vi "Main Core UI.vi"(8 "error in (no error)":errorcluster, 11 "Module_Refs":T5={"ModuleName"=enum."Controller", "Queue"=refnum, "user event"=refnum, "VI Refnum"=refnum, "ShowFP"=FALSE, "StatesTracking Enabled"=FALSE}) -> (0 "error out":errorcluster)   [LabVIEW 2021, in "Core UI.lvlib"]
doc: "Main Module Template of the architecture. Use this as a template to integrate new independent processes into your application."
uses:
  Core UI.lvlib
  Typedefs/Module References.ctl
  Typedefs/Enum_Module_Name.ctl
  Typedefs/Message.ctl
  GameEl_class/private/Enum Direction.ctl
  Application/Backgroud_v2.ctl
  Application/Shield.ctl
  Application/Grapes.ctl
  Typedefs/State Machine Data.ctl
  Typedefs/Config.ctl
  Configuration/Typedefs/App Cfg DVR.ctl
  Typedefs/Application Configuration.ctl
  Module Template/Typedefs/Config.ctl
  Modules/Sound Manager/Typedefs/Config.ctl
  Core UI Configuraton Extractor API.vi
  Configuration/Configuration.lvlib
  Architecture.lvlib
  Module Template/Module Template.lvlib
  Modules/Sound Manager/Sound Manager.lvlib
  GameEl_class/GameEl.lvclass
  Application/Application.lvclass
panel:
  out "Image Ring":u16(ring)
  out "Star":bool
  in  "Grapes":T1
  in  "Shield":T2
  in  "Studios":bool caption="Creator 2"
  in  "Creator":bool
  out "TIME":string
  out "SCORE":string
  out "Board Game":u32[][](array[colorbox])
  out "Background":T3=1
  in  "Usert Stop Game":bool
  in  "Pause/Resume":bool
  out "Direction":T4
  out "Current Score":u16
  in  "Stop App":bool
  out "Message":string
  in  "Stop Module":bool
  # "#Architecture\n\nPlace inside this box all visible data."
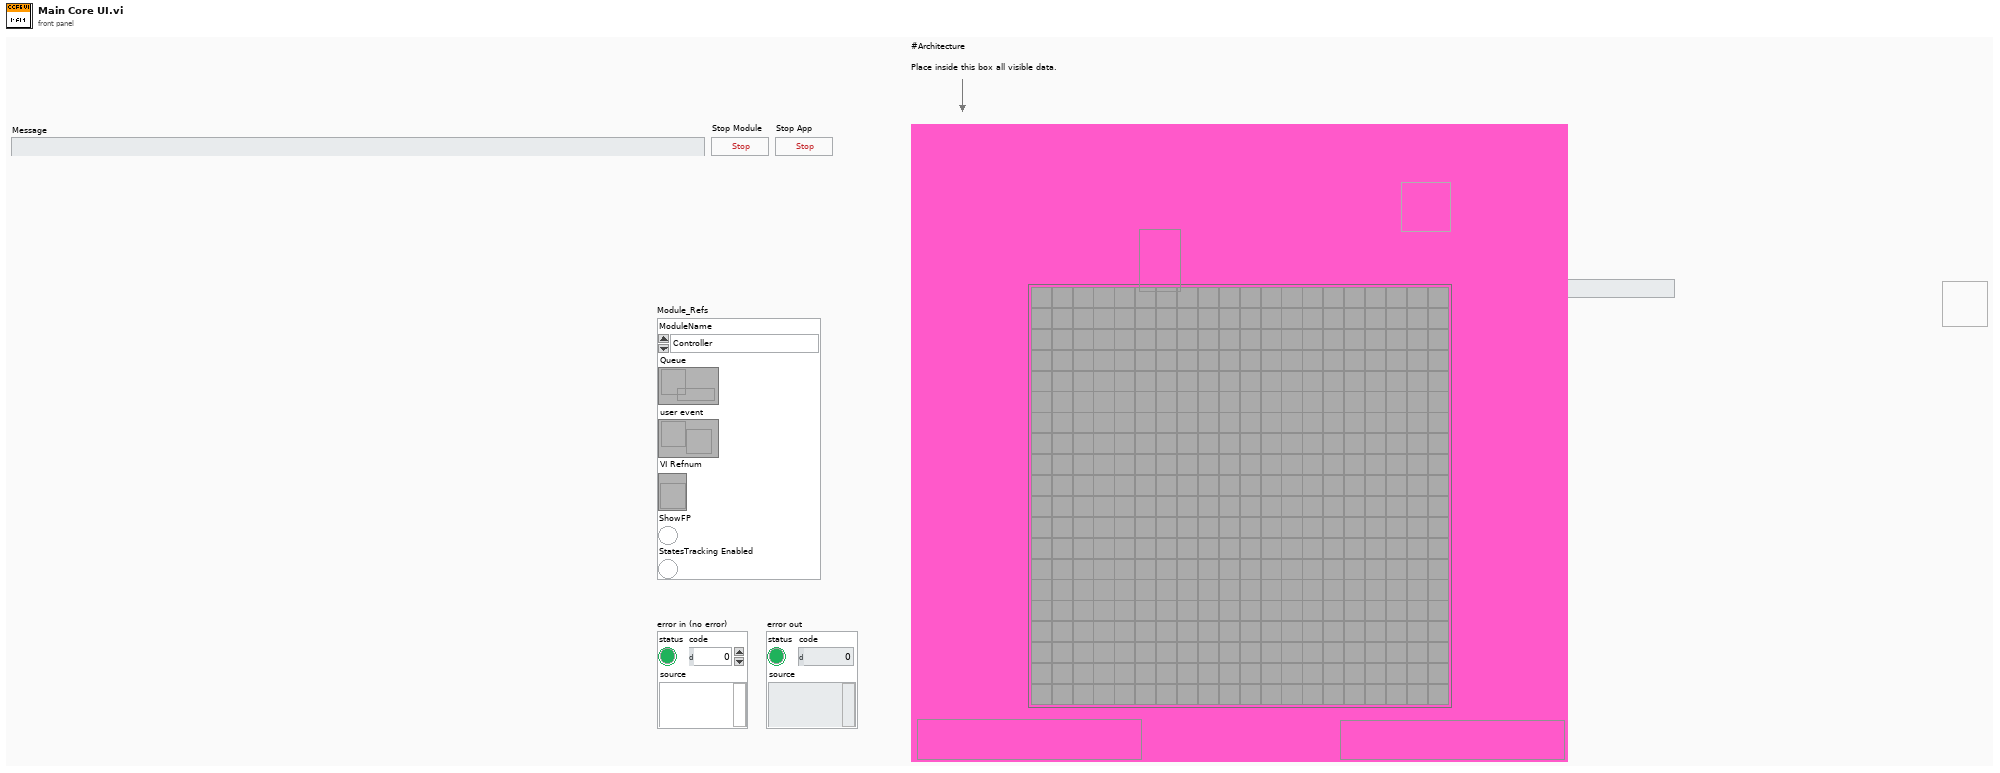
[diagram p1: front panel]
types:
  T1 = typedef "Application.lvclass/Grapes.ctl" = u16
  T2 = typedef "Application.lvclass/Shield.ctl" = u16
  T3 = typedef "Application.lvclass/Backgroud_v2.ctl" = u16
  T4 = typedef "GameEl.lvclass/Enum Direction.ctl" = enum16{"Up", "Down", "Forward", "Backward"}
  T5 = typedef "Architecture.lvlib/Module References.ctl" = cluster{"ModuleName":T6, "Queue":refnum<queue>, "user event":refnum<user-event>, "VI Refnum":refnum<vi>, "ShowFP":bool, "StatesTracking Enabled":bool}
  T6 = typedef "Configuration.lvlib/Enum_Module_Name.ctl" = enum16{"Configuration", "Error_Handler", "Log", "Database", "Controller", "UI Module", "Sound Manager"}
  T7 = typedef "Core UI.lvlib/State Machine Data.ctl" = cluster{"Module_Refs":T5, "Response Data":variant, "Core UI Config":T8}
  T8 = typedef "Core UI.lvlib/Config.ctl" = cluster{"Module Enabled":bool}
  T9 = enum32{"Invalid", "Standard", "Closed", "Hidden", "Minimized", "Maximized"}
  T10 = typedef "Error_Manager.lvlib/LogRotate.lvclass/LogData.ctl" = cluster{"error in":errorcluster, "replacements":string[], "Time Stamp":timestamp}
  T11 = typedef "Configuration.lvlib/App Cfg DVR.ctl" = refnum<data-value>
  T12 = typedef "Module Template.lvlib/Config.ctl" = cluster{"Module Enabled":bool}
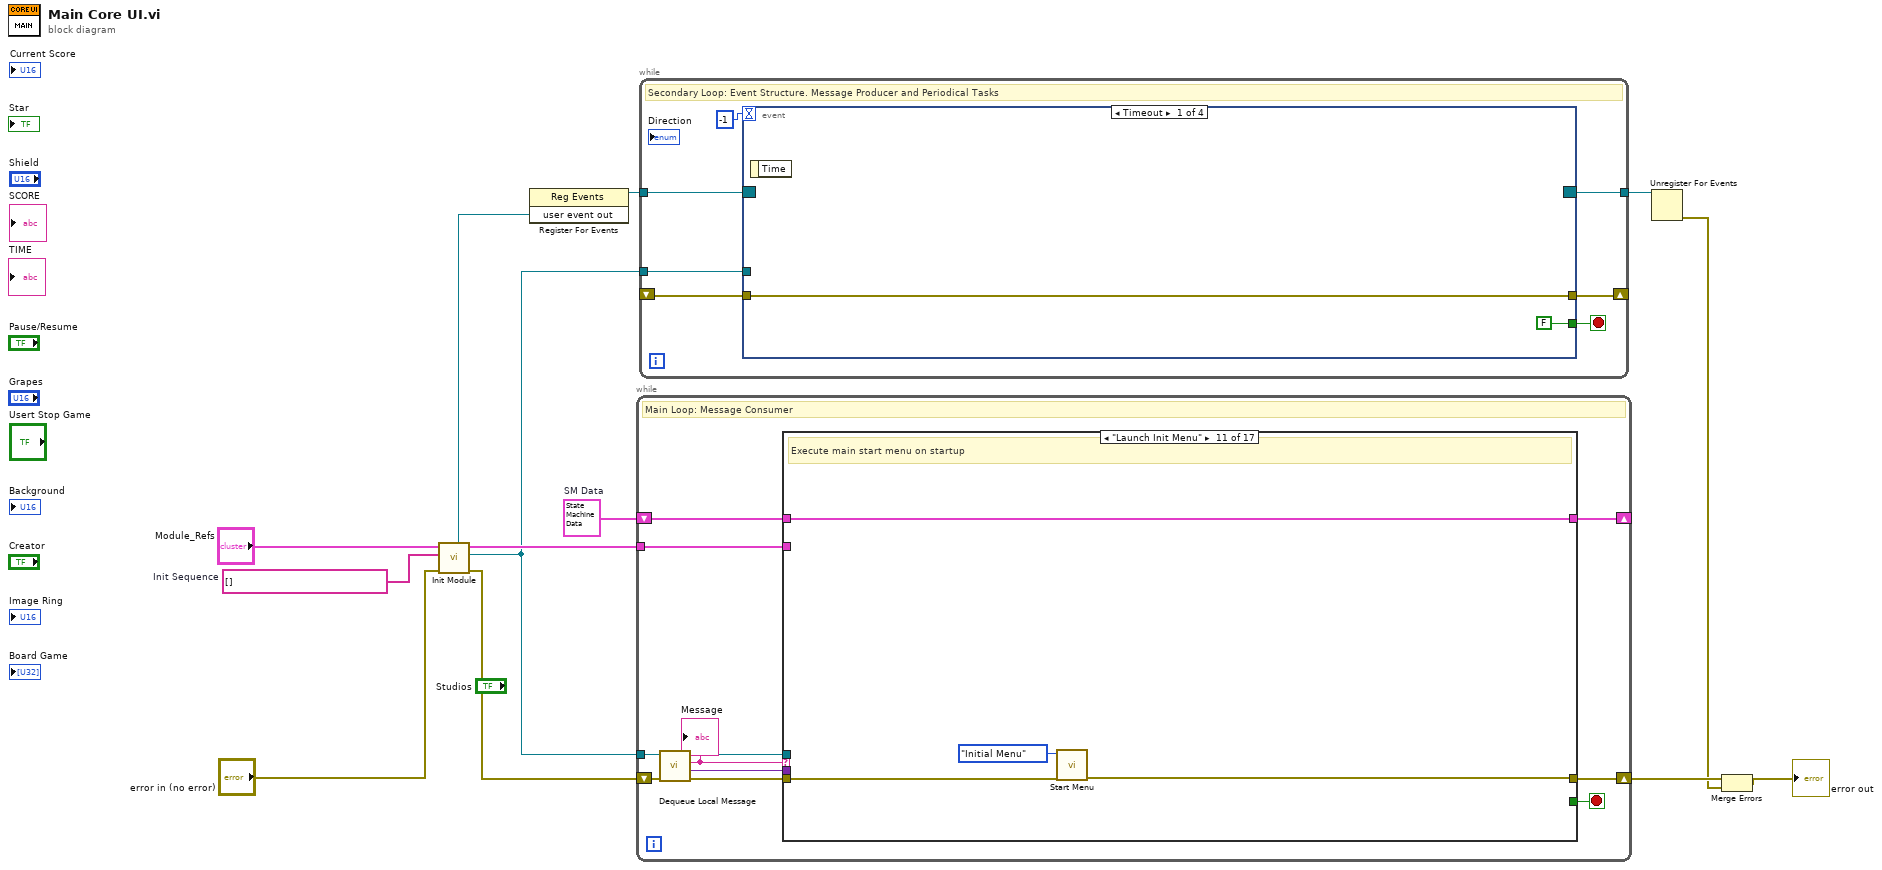
[diagram p0: block diagram]
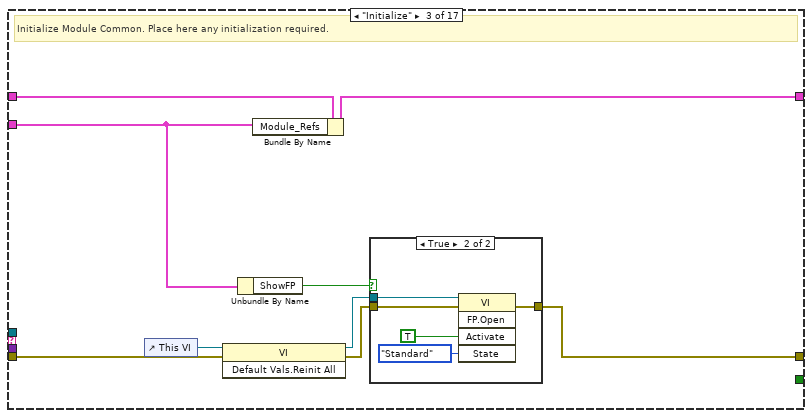
[diagram p4: hidden frame]
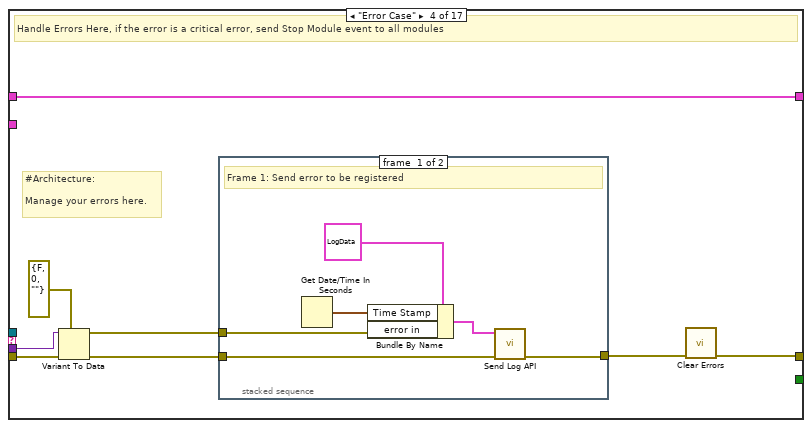
[diagram p6: hidden frame]
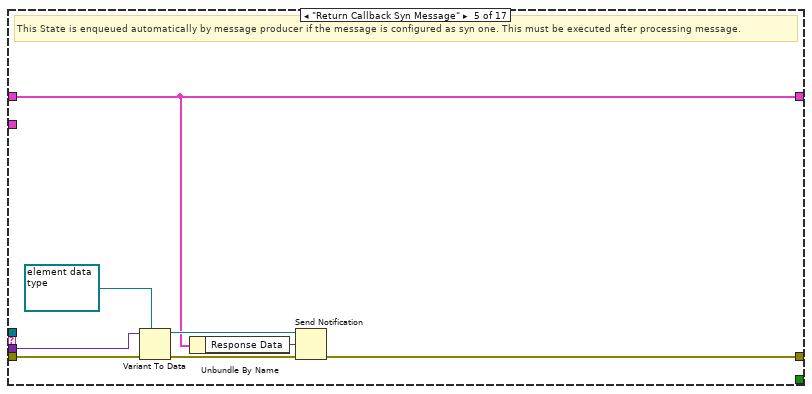
[diagram p9: hidden frame]
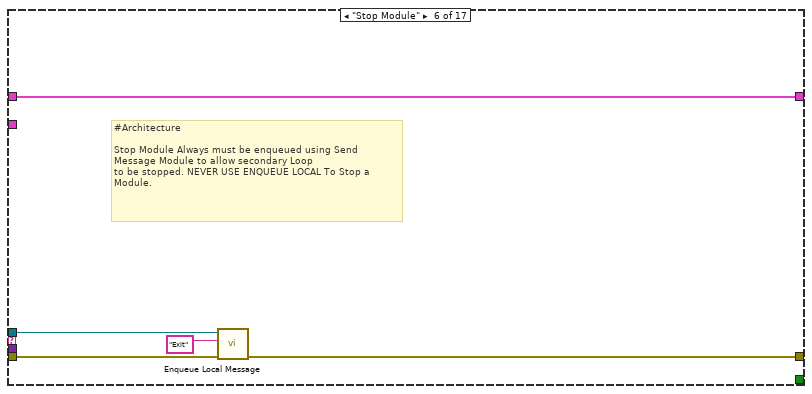
[diagram p10: hidden frame]
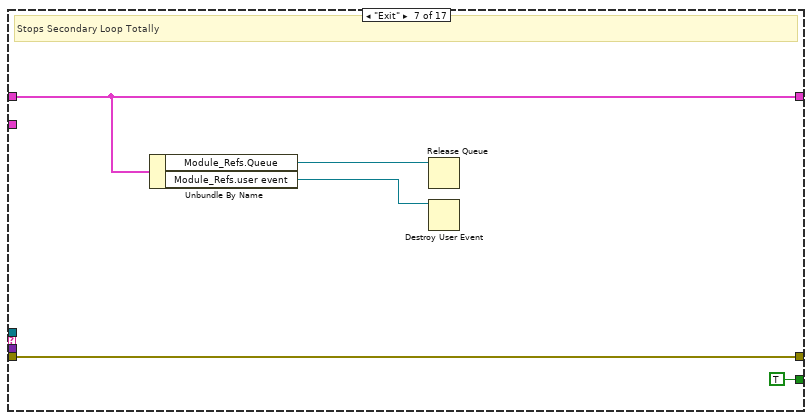
[diagram p11: hidden frame]
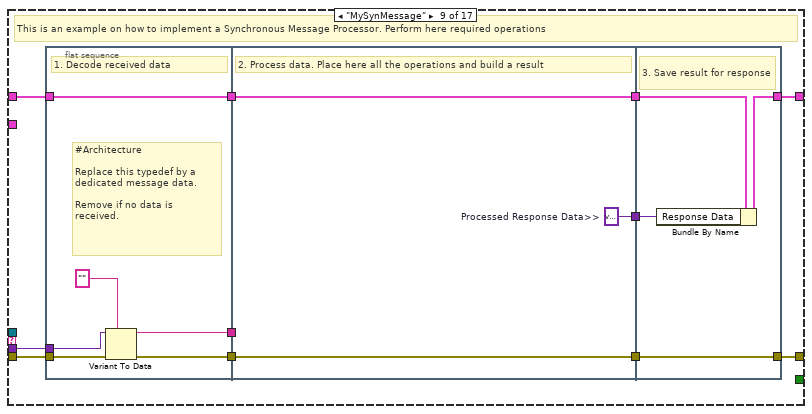
[diagram p13: hidden frame]
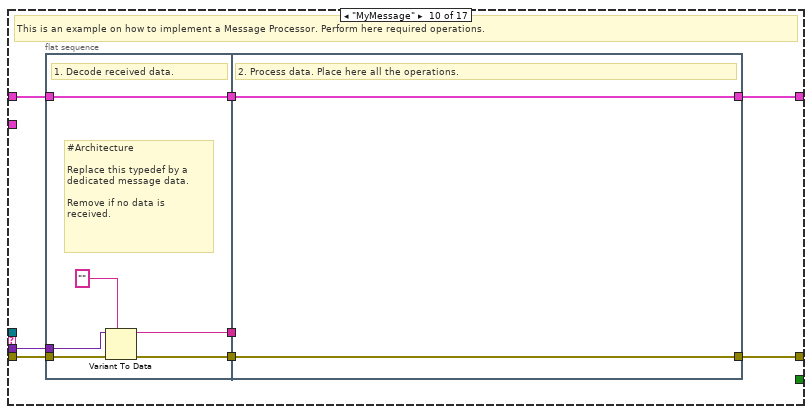
[diagram p14: hidden frame]
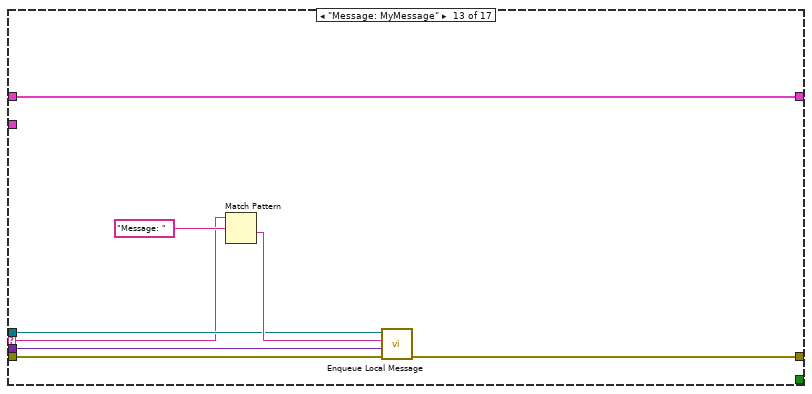
[diagram p16: hidden frame]
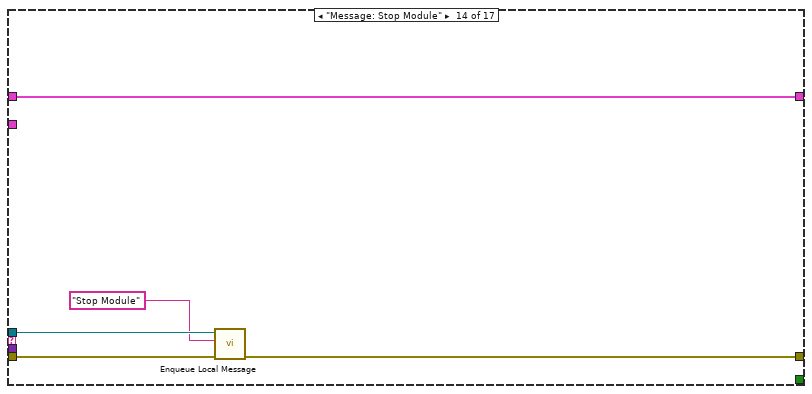
[diagram p17: hidden frame]
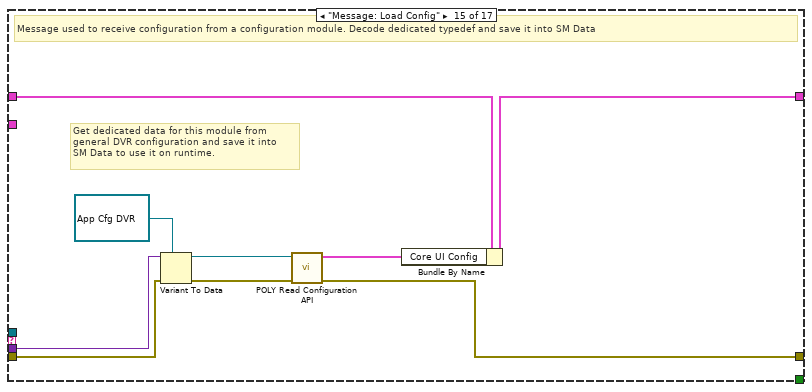
[diagram p18: hidden frame]
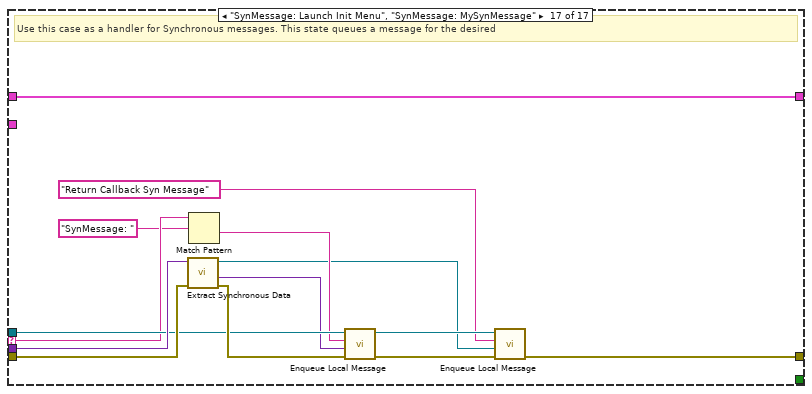
[diagram p20: hidden frame]
diagram:
  w10 = string[] []  # Init Sequence
  w13 = T7 {"Module_Refs"={"ModuleName"=enum."Controller", "Queue"=refnum, "user event"=refnum, "VI Refnum"=refnum, "ShowFP"=FALSE, "StatesTracking Enabled"=FALSE}, "Response Data"=variant, "Core UI Config"={"Module Enabled"=FALSE}}  # SM Data
  n1 = call "Init Module.vi"("error in (no error)"="error in (no error)", "Init Sequence"=w10, "Module Refs"="Module_Refs") -> ("error out"=w12:errorcluster, "queue out"=w1:refnum<queue>, "Module Refs Out"=w3:T5, "user event out"=w2:refnum<user-event>)  [unwired: 5 in]
  n2 = register-events(w2) -> (reference out=w9:refnum<event-registration>)  [unwired: 2 in, 1 out]
  n3 = while {
    shift-right: [w23] -> _
    shift-left: w13 -> [w24]
    shift-right: [w22] -> w7
    shift-left: w12 -> [w20]
    tunnel: w1 -> [w21]
    tunnel: w3 -> [w14]
    stop <- w15 stop-if-true
    # "Main Loop: Message Consumer"
    n4 = call "Dequeue Local Message.vi"("error in"=w20, "Msg queue in"=w21) -> ("error out"=w19:errorcluster, "Data"=w16:variant, "Message"=w17:string, "queue out"=w18:refnum<queue>)  [unwired: 6 in]
    "Message" <- w17
    n5 = case shown="\"Launch Init Menu\"" w17 {
      selector: w17 -> [_ _ _ _ _ _ _ _ _ _ _ _ w128 _ _ _ w160]
      tunnel: w24 -> [w26 w28 w37 w51 w63 w74 w77 w81 w92 w113 w125 w127 w135 w140 w149 w151 w165]
      tunnel: [w26 w28 w35 w51 w63 w74 w77 w81 w91 w106 w125 w127 w135 w140 w143 w151 w165] -> w23
      tunnel: w19 -> [w25 w27 w36 w50 w69 w73 w79 w80 w85 w109 w124 w126 w132 w139 w148 w150 w164]
      tunnel: [w25 w27 w31 w44 w68 w72 w79 w80 w90 w112 w123 w126 w129 w138 w144 w150 w154] -> w22
      tunnel: w18 -> [_ _ _ _ _ w71 _ _ _ _ _ _ w130 w137 _ _ w161]
      tunnel: w16 -> [_ _ _ w49 w66 _ _ _ w84 w108 _ _ w131 _ w147 _ w162]
      tunnel: [_ _ _ _ _ _ TRUE _ _ _ _ _ _ _ _ _ _] -> w15
      tunnel: w14 -> [_ _ w34 _ _ _ _ _ _ _ _ _ _ _ _ _ _]
      frame "--------State Machine Arquitechture Operations--------" {
      }
      frame "Idle", Default {
        # "Use this state to make iterations if required."
      }
      frame "Initialize" {
        # "Initialize Module Common. Place here any initialization required."
        n6 = control-ref of="This VI"() -> (w29:refnum<vi>)
        n7 = invoke class="VI" method="Default Vals.Reinit All"(reference=w29, error in=w36) -> (reference out=w32:refnum<vi>, error out=w33:errorcluster)  [unwired: 1 in, 1 out]
        n8 = Unbundle By Name(w34) -> ("ShowFP"=w30:bool)
        n9 = Bundle By Name(cluster=w37, "Module_Refs"=w34) -> (w35:T7)
        n10 = case shown="True" w30 {
          tunnel: w33 -> [w38 w43]
          tunnel: [w38 w42] -> w31
          tunnel: w32 -> [_ w41]
          frame False {
          }
          frame True {
            n11 = invoke class="VI" method="FP.Open"(reference=w41, error in=w43, "Activate"=TRUE ("Activate?"), "State"=T9."Standard") -> (error out=w42:errorcluster)  [unwired: 1 in, 4 out]
          }
        }
      }
      frame "Error Case" {
        # "#Architecture: \n\nManage your errors here."
        # "Handle Errors Here, if the error is a critical error, send Stop Module event to all modules"
        n12 = Variant To Data(error in=w50, type=errorcluster {"status"=FALSE, "code"=0, "source"=""} ("error constant"), Variant=w49) -> (data=w45:errorcluster, error out=w47:errorcluster)
        n13 = stacked-sequence {
          tunnel: w47 -> [w57 w59]
          tunnel: [w56 _] -> w46
          tunnel: w45 -> [w54 w58]
          frame #0 {
            # "Frame 1: Send error to be registered"
            n14 = Get Date/Time In Seconds() -> (seconds since 1Jan1904=w53:timestamp)
            n15 = Bundle By Name(cluster=T10 {"error in"={"status"=FALSE, "code"=0, "source"=""}, "replacements"=[], "Time Stamp"=timestamp(0 s since 1904-01-01)} ("Data"), "Time Stamp"=w53, "error in"=w54) -> (w52:T10)
            n16 = call "Send Log API.vi"("error in (no error)"=w57, "Data"=w52) -> ("error out"=w56:errorcluster)  [unwired: 9 in]
          }
          frame #1 {
            # "Frame 2: Manage your errors here"
            n17 = case shown="No Error" w58 {
              tunnel: [w60 w61] -> _
              tunnel: w59 -> [w60 w61]
              frame No Error {
              }
              frame Error {
                # "#Architecture \n\nPlace here critical errors to be managed \nin the desired way."
              }
            }
          }
        }
        n18 = call <vilib>:"Clear Errors.vi"("error in (no error)"=w46) -> ("error out"=w44:errorcluster)  [unwired: 5 in, 1 out]
      }
      frame "Return Callback Syn Message" {
        # "This State is enqueued automatically by message producer if the message is configured as syn one. This must be executed after processing message."
        n19 = Variant To Data(error in=w69, type=refnum<notifier> refnum ("notifier out"), Variant=w66) -> (data=w64:refnum<notifier>, error out=w67:errorcluster)
        n20 = Unbundle By Name(w63) -> ("Response Data"=w62:variant)
        n21 = Send Notification(notification=w62, notifier=w64, error in (no error)=w67) -> (error out=w68:errorcluster)  [unwired: 1 out]
      }
      frame "Stop Module" {
        # "#Architecture\n\nStop Module Always must be enqueued using Send Message Module to allow secondary Loop\nto be stopped. NEVER USE ENQUEUE LOCAL To Stop a Module."
        n22 = call "Enqueue Local Message.vi"("error in"=w73, "Message"="Exit", "Msg queue in"=w71) -> ("error out"=w72:errorcluster)  [unwired: 7 in, 1 out]
      }
      frame "Exit" {
        # "Stops Secondary Loop Totally"
        n23 = Unbundle By Name(w77) -> ("Module_Refs.Queue"=w76:refnum<queue>, "Module_Refs.user event"=w75:refnum<user-event>)
        n24 = Release Queue(queue=w76) -> ()  [unwired: 2 in, 3 out]
        n25 = Destroy User Event(user event=w75) -> ()  [unwired: 1 in, 1 out]
      }
      frame "--------------State Machine Custom States-------------" {
      }
      frame "MySynMessage" {
        # "This is an example on how to implement a Synchronous Message Processor. Perform here required operations"
        n26 = flat-sequence {
          tunnel: w85 -> [w96]
          tunnel: w92 -> [w98]
          tunnel: [w98] -> w89
          tunnel: [w94] -> w88
          tunnel: w84 -> [w95]
          tunnel: [w93] -> w83
          tunnel: w89 -> [w101]
          tunnel: w88 -> [w100]
          tunnel: [w101] -> w87
          tunnel: [w100] -> w86
          tunnel: w83 -> [_]
          tunnel: [w99] -> w82
          tunnel: [w104] -> w90
          tunnel: [w103] -> w91
          tunnel: w87 -> [w105]
          tunnel: w86 -> [w104]
          tunnel: w82 -> [w102]
          frame #0 {
            # "#Architecture\n\nReplace this typedef by a dedicated message data.\n\nRemove if no data is received."
            # "1. Decode received data"
            n27 = Variant To Data(error in=w96, type="", Variant=w95) -> (data=w93:string, error out=w94:errorcluster)
          }
          frame #1 {
            w99 = variant  # Processed Response Data>>
            # "2. Process data. Place here all the operations and build a result"
          }
          frame #2 {
            # "3. Save result for response"
            n28 = Bundle By Name(cluster=w105, "Response Data"=w102) -> (w103:T7)
          }
        }
      }
      frame "MyMessage" {
        # "This is an example on how to implement a Message Processor. Perform here required operations."
        n29 = flat-sequence {
          tunnel: w109 -> [w117]
          tunnel: w113 -> [w119]
          tunnel: [w119] -> w111
          tunnel: [w115] -> w110
          tunnel: w108 -> [w116]
          tunnel: [w114] -> w107
          tunnel: w111 -> [w120]
          tunnel: w110 -> [w121]
          tunnel: w107 -> [_]
          tunnel: [w121] -> w112
          tunnel: [w120] -> w106
          frame #0 {
            # "#Architecture\n\nReplace this typedef by a dedicated message data.\n\nRemove if no data is received."
            # "1. Decode received data."
            n30 = Variant To Data(error in=w117, type="", Variant=w116) -> (data=w114:string, error out=w115:errorcluster)
          }
          frame #1 {
            # "2. Process data. Place here all the operations."
          }
        }
      }
      frame "Launch Init Menu" {
        # "Execute main start menu on startup"
        n31 = call "Start Menu.vi"("error in (no error)"=w124, "Enum"=enum16{"Initial Menu", "Final Menu"}."Initial Menu") -> ("error out"=w123:errorcluster)  [unwired: 9 in]
      }
      frame "--------------Dynamic Events Messages----------------" {
      }
      frame "Message: MyMessage" {
        n32 = Match Pattern(string=w128, regular expression="Message: ") -> (after substring=w133:string)  [unwired: 1 in, 3 out]
        n33 = call "Enqueue Local Message.vi"("error in"=w132, "Data"=w131, "Message"=w133, "Msg queue in"=w130) -> ("error out"=w129:errorcluster)  [unwired: 6 in, 1 out]
      }
      frame "Message: Stop Module" {
        n34 = call "Enqueue Local Message.vi"("error in"=w139, "Message"="Stop Module", "Msg queue in"=w137) -> ("error out"=w138:errorcluster)  [unwired: 7 in, 1 out]
      }
      frame "Message: Load Config" {
        # "Get dedicated data for this module from \ngeneral DVR configuration and save it into \nSM Data to use it on runtime."
        # "Message used to receive configuration from a configuration module. Decode dedicated typedef and save it into SM Data"
        n35 = Variant To Data(error in=w148, type=T11 refnum ("App Cfg DVR"), Variant=w147) -> (data=w146:T11, error out=w145:errorcluster)
        n36 = call-poly "POLY Read Configuration API.vi"("error constant"=w145, "App Cfg DVR"=w146) -> ("error out"=w144:errorcluster, "Module Template Config"=w142:T12)  [unwired: 8 in]
        n37 = Bundle By Name(cluster=w149, "Core UI Config"=w142) -> (w143:T7)
      }
      frame "------------Synchronous Event Messages--------------" {
      }
      frame "SynMessage: Launch Init Menu", "SynMessage: MySynMessage" {
        # "Use this case as a handler for Synchronous messages. This state queues a message for the desired"
        n38 = call "Extract Synchronous Data.vi"("error in 2"=w164, "Variant"=w162) -> ("error in"=w163:errorcluster, "Data Out"=w157:variant, "notifier out"=w152:refnum<notifier>)  [unwired: 7 in]
        n39 = Match Pattern(string=w160, regular expression="SynMessage: ") -> (after substring=w158:string)  [unwired: 1 in, 3 out]
        n40 = call "Enqueue Local Message.vi"("error in"=w163, "Data"=w157, "Message"=w158, "Msg queue in"=w161) -> ("error out"=w156:errorcluster, "queue out"=w155:refnum<queue>)  [unwired: 6 in]
        n41 = call "Enqueue Local Message.vi"("error in"=w156, "Data"=w152, "Message"="Return Callback Syn Message", "Msg queue in"=w155) -> ("error out"=w154:errorcluster)  [unwired: 6 in, 1 out]
      }
    }
  }
  n42 = while {
    tunnel: w9 -> [w172]
    tunnel: w1 -> [w169]
    tunnel: [w168] -> w8
    shift-right: [w166] -> _
    shift-left: _ -> [w167]
    stop <- w170 stop-if-true
    # "Secondary Loop: Event Structure. Message Producer and Periodical Tasks"
    n43 = event shown="[0] Timeout" {
      selector: w172 -> [_ _ _ _]
      dyn-events: [_ _ _ _] -> w168
      timeout: -1 -> [_ _ _ _]
      tunnel: [FALSE w181 TRUE _] -> w170
      tunnel: w169 -> [_ w186 w188 _]
      tunnel: w167 -> [w173 w185 w191 w193]
      tunnel: [w173 w184 w189 w192] -> w166
      event Timeout {
        n44 = event-data() -> ()  [unwired: 1 in, 1 out]
      }
      event User Event {
        # "Send message to local queue. \n(Message Consumer)"
        # "Processes an external event and enqueues a message to the local queue. It can be synchronous (with response) or NOT."
        n45 = event-data() -> ("syn"=w178:bool, "Message"=w180:string, "Data"=w183:variant)  [unwired: 1 in]
        n46 = Select(t="SynMessage: " ("string"), s=w178, f="Message: " ("string")) -> (s? t:f=w175:string)
        n47 = Concatenate Strings(w175, w180) -> (w182:string)
        n48 = call "Enqueue Local Message.vi"("error in"=w185, "Data"=w183, "Message"=w182, "Msg queue in"=w186) -> ("error out"=w184:errorcluster)  [unwired: 6 in, 1 out]
        n49 = Equal?(x=w180, y="Stop Module") -> (x = y?=w181:bool)
      }
      event "Stop Module": Value Change {
        n50 = event-data() -> ()  [unwired: 1 in, 1 out]
        n51 = call "Enqueue Local Message.vi"("error in"=w191, "Message"="Stop Module", "Msg queue in"=w188) -> ("error out"=w189:errorcluster)  [unwired: 7 in, 1 out]
      }
      event "Stop App": Value Change {
        w195 = TRUE  # All Modules
        # "Send Stop To All Modules"
        n52 = event-data() -> ()  [unwired: 1 in, 1 out]
        n53 = call "Send Message Modules.vi"("All Modules"=w195, "Error In"=w193, "Message"="Stop Module") -> ("error in (no error)"=w192:errorcluster)  [unwired: 8 in]
      }
    }
  }
  n54 = Unregister For Events(event registration refnum=w8) -> (error out=w6:errorcluster)  [unwired: 1 in]
  n55 = Merge Errors(w7, w6) -> (→"error out":errorcluster)
